vi "Untitled 35.vi"() -> ()   [LabVIEW 2013]
uses:
  <vilib>/addons/control/pid/NI_PID_pid.lvlib
  <vilib>/addons/control/pid/pid.llb/PID Control Input Filter (DBL).vi
  <vilib>/Simulation/Implementation/Shared/SIMSCR Execution Mode.ctl
  <vilib>/Simulation/Scripting/Companion Diagram/SimConfigNode/_simSolvers.ctl
  <vilib>/Simulation/Scripting/Companion Diagram/SimConfigNode/SimParams.ctl
  <vilib>/Simulation/Scripting/Companion Diagram/SimConfigNode/SimDog.xnode
  <vilib>/Simulation/Implementation/XNodeFramework/SimXNode/SimX.xnode
  Input.vi
  LinearControl.vi
panel:
  out "Boolean":bool
  out "stop_1":bool
  in  "start":bool
  in  "stop":bool
  in  "Enable":bool
  in  "res_pos_X":bool
  out "pos_X":dbl
  in  "res_theta":bool
  out "theta":dbl
  out "x_e":dbl
  out "xdot_e":dbl
  out "theta_e":dbl
  out "thetadot_e":dbl
  in  "setpoint":dbl
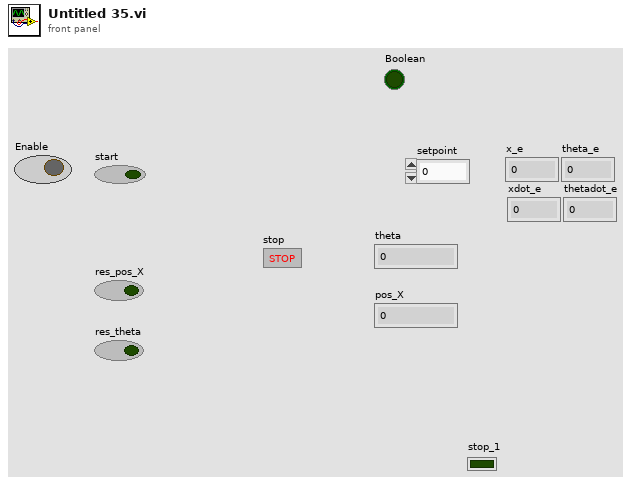
[diagram p1: front panel]
types:
  T1 = enum16{"Simulate to Completion", "Single Time-Step Simulation (Fixed Step Only)"}
  T2 = typedef "SimParams.ctl" = cluster{"Initial Time (s)":dbl, "Final Time (s)":dbl, "Step Size (s)":dbl, "ODE Solver":T3, "Minimum Step Size (s)":dbl, "Maximum Step Size (s)":dbl, "Relative Tolerance":dbl, "Absolute Tolerance":dbl, "Software Timing":bool, "Initial Step Size (s)":dbl, "Automatic Fixed Step Size?":bool, "Automatic Discrete Step Size?":bool, "Discrete Step Size (s)":dbl, "Calculate using Time Step":bool, "Solver Wired?":bool, "Prev.Frm.Expected End":u64, "Prev.Frm.Actual End":u64, "Prev.Frm.Finished Late?":bool, "Prev.Iter.Expected End":u64, "Prev.Iter.Actual End":u64, "Prev.Iter.Finished Late?":bool, "Expected Iteration Start":u64, "Actual Iteration Start":u64, "Expected Frame Start":u64, "Actual Frame Start":u64, "Source Name":string, "Name":string, "Period":i64, "Deadline":i64, "Offset":i64, "Start":i64, "Priority":i32, "Timeout":i32, "Processor":i32, "Mode":enum32{"No Change", "Process missed periods, maintain original phase", "Discard missed periods, maintain original phase", "Process missed periods, ignore original phase", "Discard missed periods, ignore original phase"}, "Wakeup reason":enum32{"Normal", "Aborted", "Asynchronous wakeup", "Timing source error", "Timed loop error", "Timeout"}, "Error":errorcluster, "Source Type":string, "Secondary Source Type":string, "Global End Time":u64, "Global Start Time":u64, "Full Solver Reset":bool, "Execution Mode":T4, "Nan/Inf Check":bool, "Custom Solver Library":string, "Solver Is Variable":bool, "custom solver name":string, "Signal Collection Decimation":u32}
  T3 = typedef "_simSolvers.ctl" = enum16{"Runge-Kutta 1 (Euler)", "Runge-Kutta 2", "Runge-Kutta 3", "Runge-Kutta 4", "Runge-Kutta 23 (variable)", "Runge-Kutta 45 (variable)", "BDF (variable)", "Adams-Moulton (variable)", "Rosenbrock (variable)", "Discrete States Only", "SDIRK 4 (variable)", "Radau 5 (variable)", "Radau 9 (variable)", "Radau 13 (variable)", "Radau [Variable Order] (variable)", "Gear's Method (variable)", "Linearizer", "State Query", "Trim Eval", "Custom Solver"}
  T4 = typedef "SIMSCR Execution Mode.ctl" = enum16{"Simulate to Completion", "Single Time-Step Simulation (Fixed Step Only)"}
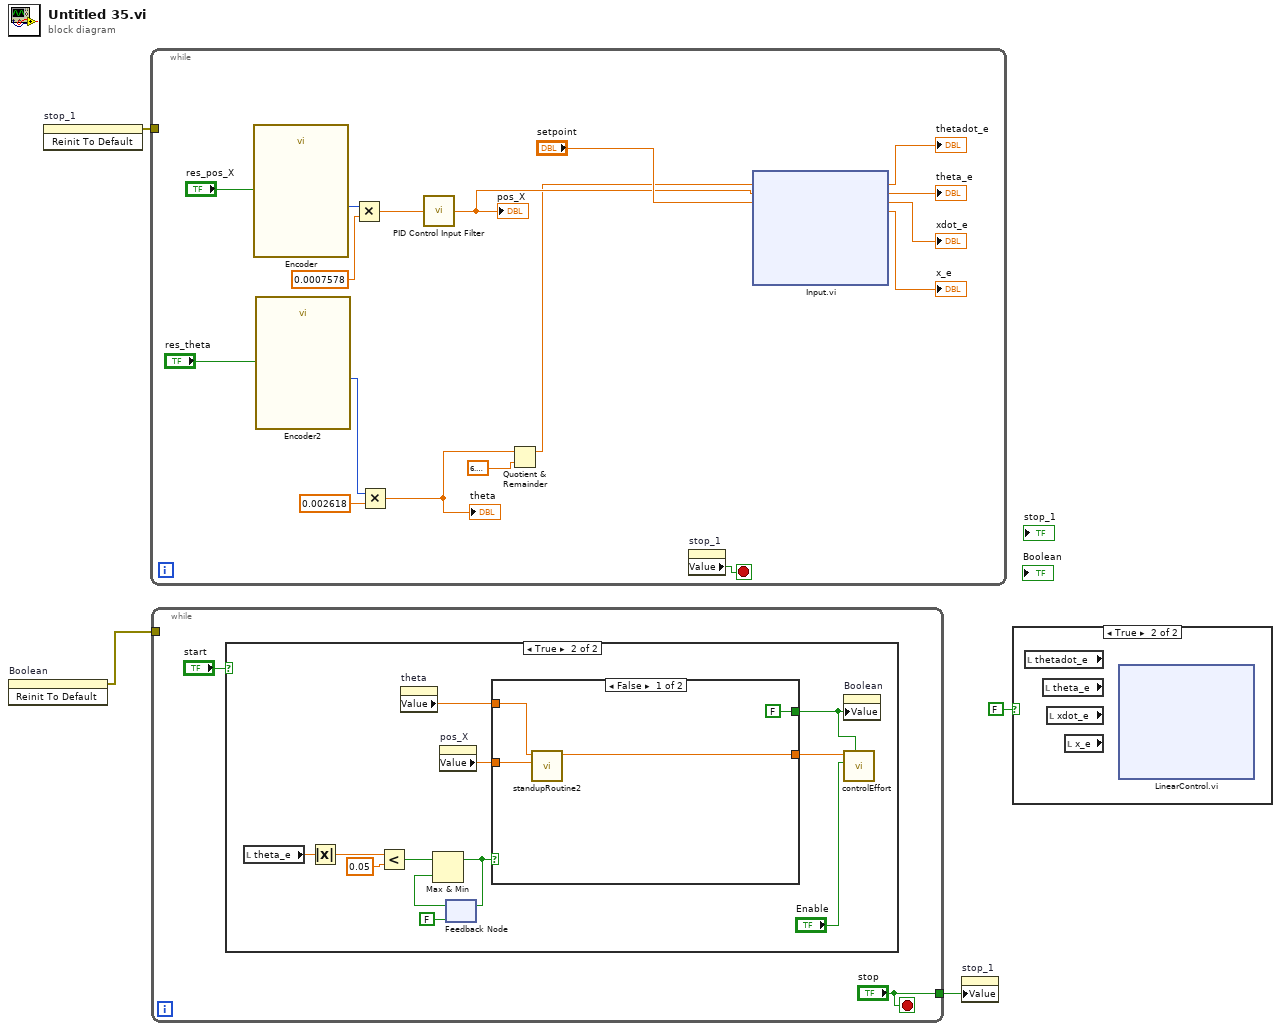
[diagram p0: block diagram]
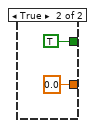
[diagram p4: hidden frame]
diagram:
  n1 = invoke on="Boolean" class="Bool (strict)" method="Reinit To Default"() -> (error out=w2:errorcluster)  [unwired: 3 in, 2 out]
  n2 = invoke on="stop_1" class="Bool (strict)" method="Reinit To Default"() -> (error out=w3:errorcluster)  [unwired: 3 in, 2 out]
  n3 = while {
    tunnel: w3 -> [_]
    stop <- w15 stop-if-true
    n4 = call "Encoder"("Reset Counter"="res_pos_X") -> ("Counter Value"=w20:i32)  [unwired: 23 in, 3 out]
    n5 = call "Encoder2"("Reset Counter"="res_theta") -> ("Counter Value"=w17:i32)  [unwired: 23 in, 3 out]
    n6 = Multiply(x=w20, y=0.0007578 ("y 2")) -> (x*y=w18:dbl)
    n7 = Multiply ("Multiply 2")(x=w17, y=0.002618) -> (x*y=w5:dbl)
    "theta" <- w5
    n8 = call-poly <vilib>:"PID Control Input Filter.vi"("input"=w18) -> ("output"=w13:dbl)  [unwired: 4 in]
    "pos_X" <- w13
    n9 = Quotient & Remainder(x=w5, y=6.283185307179586 ("Constant")) -> (x-y*floor(x/y)=w6:dbl)  [unwired: 1 out]
    n10 = property on="stop_1" class="Bool (strict)"() -> ("Value"=w15:bool)  [unwired: 2 in, 2 out]
    n11 = xnode "Input.vi"("theta"=w6, "x"=w13, "setpoint"="setpoint") -> ("thetadot_e"=→"thetadot_e":dbl, "theta_e"=→"theta_e":dbl, "xdot_e"=→"xdot_e":dbl, "x_e"=→"x_e":dbl)  [unwired: 2 in, 6 out]
  }
  n12 = while {
    tunnel: ["stop"] -> w4
    tunnel: w2 -> [_]
    stop <- "stop" stop-if-true
    n13 = case shown="True" "start" {
      frame False {
      }
      frame True {
        n14 = local read "theta_e"() -> (w61:dbl)
        n15 = Absolute Value(x=w61) -> (abs(x)=w70:dbl)
        n16 = Less?(x=w70, y=0.05) -> (x < y?=w68:bool)
        n17 = property on="theta" class="DigNum (strict)"() -> ("Value"=w64:dbl)  [unwired: 2 in, 2 out]
        n18 = property on="pos_X" class="DigNum (strict)"() -> ("Value"=w63:dbl)  [unwired: 2 in, 2 out]
        n19 = feedback #1(FALSE) -> (w67:bool)
        n20 = Max & Min(x=w68, y=w67) -> (max(x,y)=w65:bool)  [unwired: 1 out]
        n21 = feedback-in #1(w65) -> ()
        n22 = case shown="False" w65 {
          tunnel: [w74 0.0 ("force")] -> w60
          tunnel: [FALSE TRUE] -> w62
          tunnel: w64 -> [w73 _]
          tunnel: w63 -> [w72 _]
          frame False {
            n23 = call "standupRoutine2.vi"("x"=w72, "theta"=w73) -> ("force"=w74:dbl)  [unwired: 9 in]
          }
          frame True {
          }
        }
        n24 = property on="Boolean" class="Bool (strict)"("Value"=w62) -> ()  [unwired: 2 in, 2 out]
        n25 = call "controlEffort.vi"("Inverted?"=w62, "Enable"="Enable", "force"=w60) -> ()  [unwired: 9 in]
      }
    }
  }
  n26 = property on="stop_1" class="Bool (strict)"("Value"=w4) -> ()  [unwired: 2 in, 2 out]
  n27 = case shown="True" FALSE {
    frame False {
    }
    frame True {
      n28 = local read "thetadot_e"() -> (w78:dbl)
      n29 = local read "theta_e"() -> (w79:dbl)
      n30 = local read "xdot_e"() -> (w80:dbl)
      n31 = local read "x_e"() -> (w81:dbl)
      n32 = xnode "LinearControl.vi"() -> ()  [unwired: 5 in, 9 out]
    }
  }
